vi "KH7008 Open.vi"(8 "error in (no error)":errorcluster) -> (0 "error out":errorcluster, 1 "Model":string, 2 "Serial Number":string, 3 "VISA Ref Out":refnum<visa-resource-name>)   [LabVIEW 2019, in "Inst.Krohn-Hite-7008.lvclass"]
uses:
  Inst.Krohn-Hite-7008.lvclass
  <vilib>/Instr/_visa.llb/VISA Configure Serial Port (Instr).vi
  <userlib>/LevyLab/D2XX-LV/D2XX-lv.lvlib
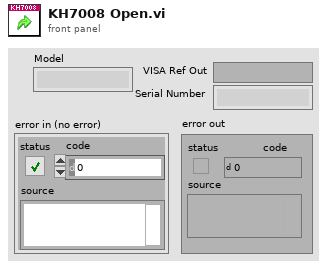
[diagram p1: front panel]
types:
  T1 = typedef "D2XX-lv.lvlib/Device Info.ctl" = cluster{"Serial Number":string, "COM port":string, "Description":string}
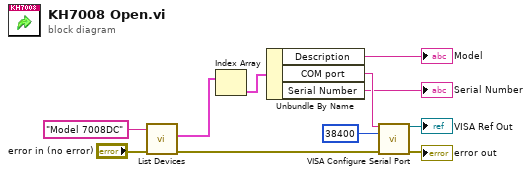
[diagram p0: block diagram]
diagram:
  n1 = call <userlib>:"List Devices.vi"("error in (no error)"="error in (no error)", "Filter (Device Description)"="Model 7008DC") -> ("error out"=w9:errorcluster, "Devices"=w7:T1[])  [unwired: 8 in]
  n2 = Index Array(array=w7) -> (element=w6:T1)  [unwired: 1 in]
  n3 = Unbundle By Name(w6) -> ("Description"=→"Model":string, "COM port"=w5:string, "Serial Number"=→"Serial Number":string)
  n4 = call-poly "VISA Configure Serial Port"("VISA resource name"=w5, "baud rate (9600)"=u32 38400, "error in (no error)"=w9) -> ("VISA resource name out"=→"VISA Ref Out":refnum<visa-resource-name>, "error out"=→"error out":errorcluster)  [unwired: 6 in, 5 out]
